vi "Main.vi"(11 "Module Admin":refnum<class "Delacor_lib_QMH_Module Admin.lvclass">) -> ()   [LabVIEW 2019, in "SME_Report.lvlib"]
doc: "This Module has below functionality.\nyou can load the csv logfile you created in the last\nstep and make the following calculations: maximum viscosity, minimum viscosity,\naverage viscosity, standard deviation of the viscosity"
uses:
  SME_Report.lvlib
  <vilib>/Delacor/Delacor QMH/Libraries/Module Admin_class/Delacor_lib_QMH_Module Admin.lvclass
  Module Data--cluster.ctl
  <vilib>/Delacor/Delacor QMH/Libraries/Message Queue_class/Delacor_lib_QMH_Message Queue.lvclass/Delacor_lib_QMH_Message Queue.ctl
  Stop Argument--cluster.ctl
  <vilib>/Delacor/Delacor QMH/Libraries/Module Admin_class/Delacor_lib_QMH_Module Admin.lvclass/Delacor_lib_QMH_Module Admin.ctl
  <vilib>/Delacor/Delacor QMH/Libraries/Message Queue_class/Delacor_lib_QMH_Enqueue Message (Single).vi
  <vilib>/Delacor/Delacor QMH/Libraries/Module Admin_class/Delacor_lib_QMH_Get External Launch.vi
  <vilib>/Delacor/Delacor QMH/Libraries/Message Queue_class/Delacor_lib_QMH_Message Queue.lvclass
panel:
  in  "Close":bool
  out "Calculation":T1 {"SD" format="%.3f"; "AVG" format="%.3f"; "Min" format="%.3f"; "Max" format="%.3f"}
  in  "Calc":bool
  in  "Path":path caption="File Path"
  out "error out":errorcluster
  out "Status":string
  in  "Simulate MHL Error":bool
  in  "Simulate EHL Error":bool
  # "Data Analysis"
  # "Other processes communicate with this Module via its Public API (wrappers for its Request Events).\n\nThis Module communicates with other processes via its Broadcast Events.\nAny process that wants to receive these messages can register for this module's Broadcast events."
  # "This template is for the DQMH framework. See the block diagram for more information on how to use this template."
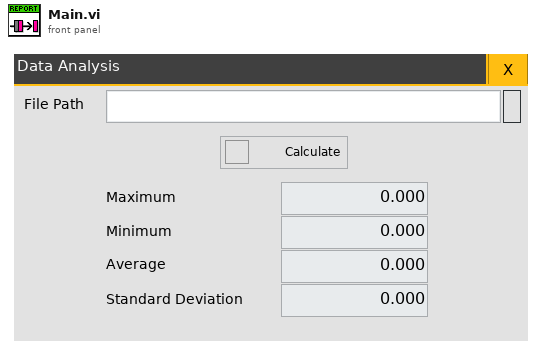
[diagram p1: front panel]
types:
  T1 = cluster{"Max":dbl, "Min":dbl, "AVG":dbl, "SD":dbl}
  T2 = typedef "SME_Report.lvlib/Request Events--cluster.ctl" = cluster{"Stop Module":refnum<user-event>, "Show Panel":refnum<user-event>, "Hide Panel":refnum<user-event>, "Get Module Execution Status":refnum<user-event>, "Show Diagram":refnum<user-event>}
  T3 = typedef "SME_Report.lvlib/Module Data--cluster.ctl" = cluster{"Status":string}
  T4 = enum32{"invalid lock state", "Not Locked", "Locked (No Password)", "Password-protected"}
  T5 = typedef "SME_Report.lvlib/Stop Argument--cluster.ctl" = cluster{"Origin":string, "Exit via Stop Module Req?":bool, "Wait for Module to stop?":bool}
  T6 = enum32{"Invalid", "Standard", "Closed", "Hidden", "Minimized", "Maximized"}
  T7 = cluster{"[0]":dbl, "[1]":dbl, "[2]":dbl, "[3]":dbl}
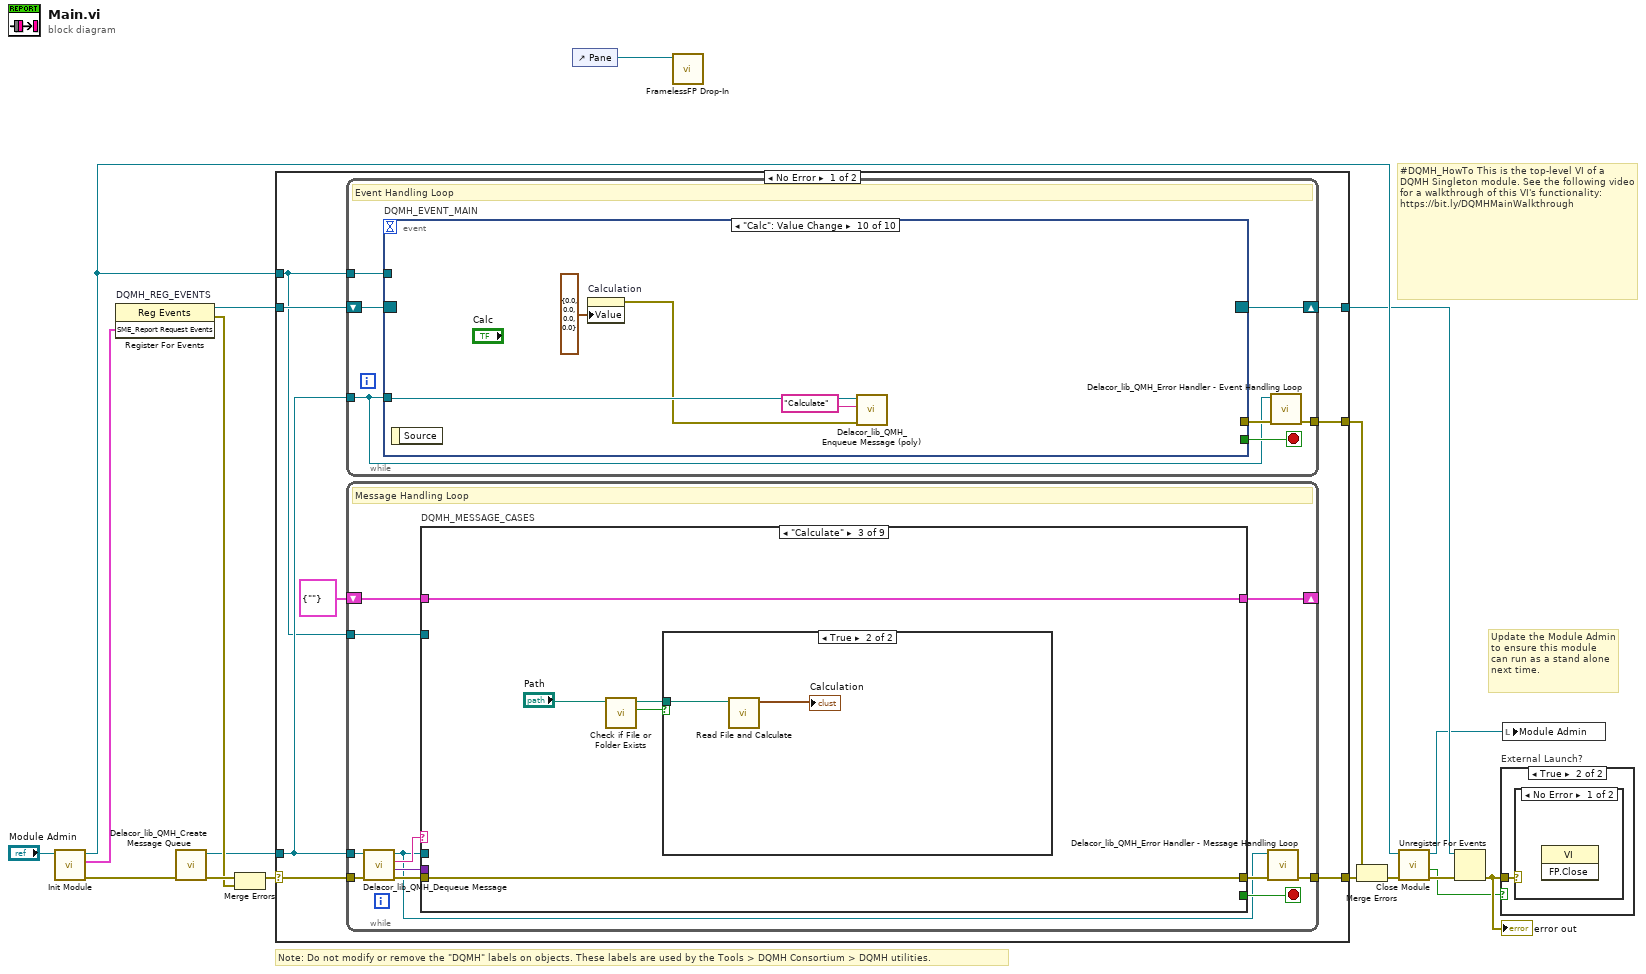
[diagram p0: block diagram]
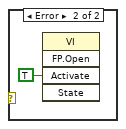
[diagram p3: hidden frame]
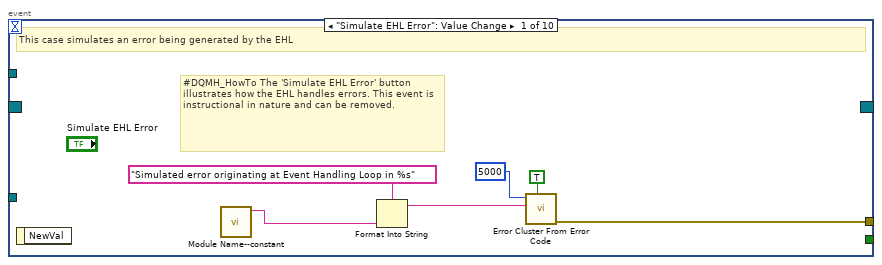
[diagram p4: hidden frame]
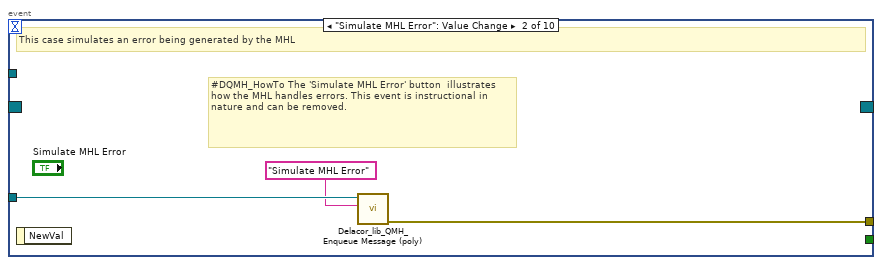
[diagram p5: hidden frame]
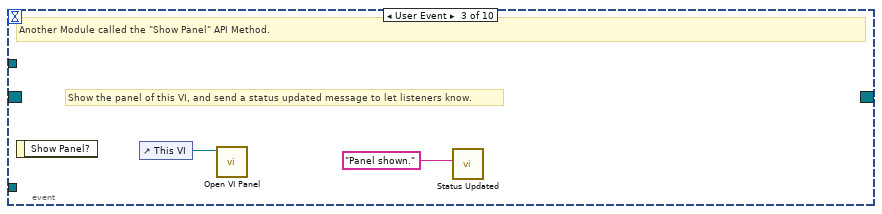
[diagram p6: hidden frame]
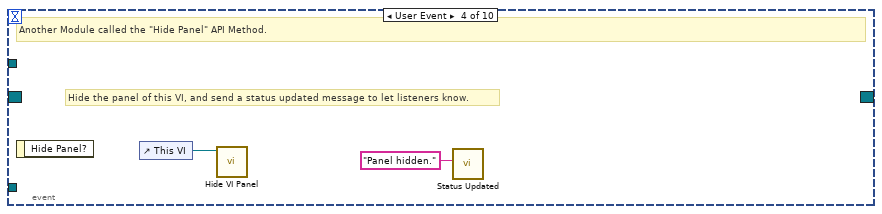
[diagram p7: hidden frame]
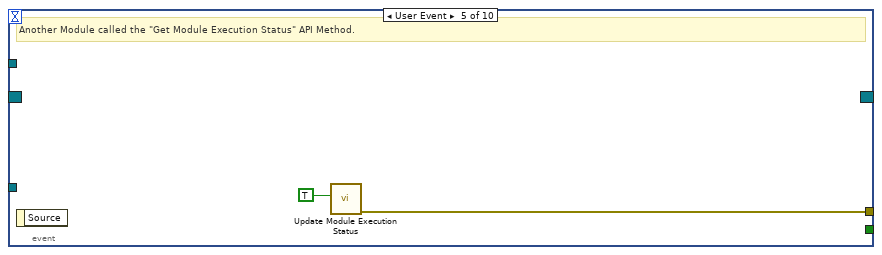
[diagram p8: hidden frame]
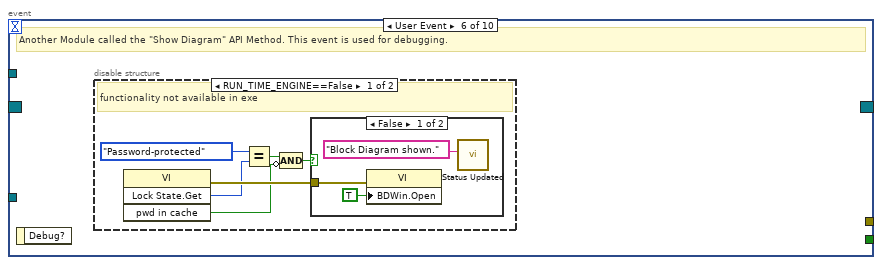
[diagram p9: hidden frame]
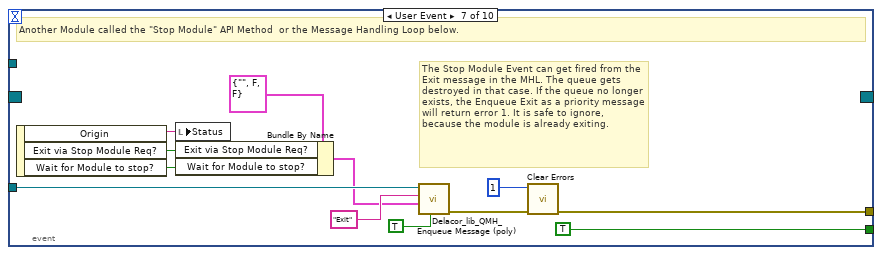
[diagram p12: hidden frame]
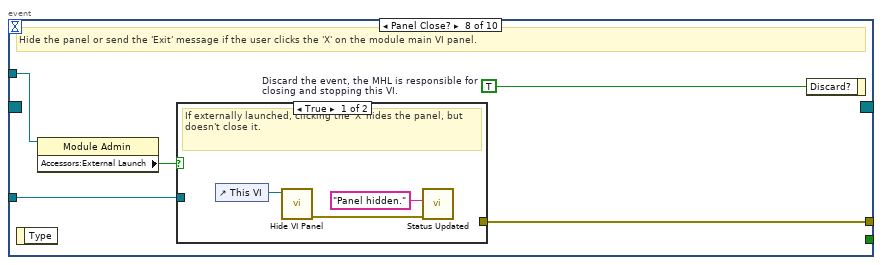
[diagram p13: hidden frame]
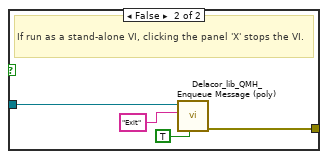
[diagram p14: hidden frame]
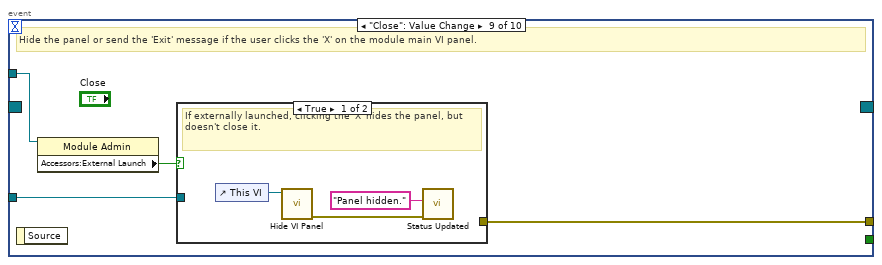
[diagram p15: hidden frame]
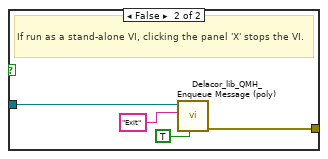
[diagram p16: hidden frame]
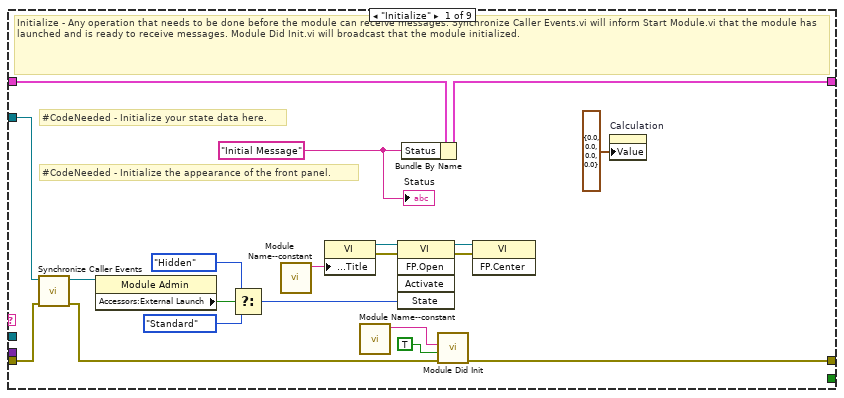
[diagram p17: hidden frame]
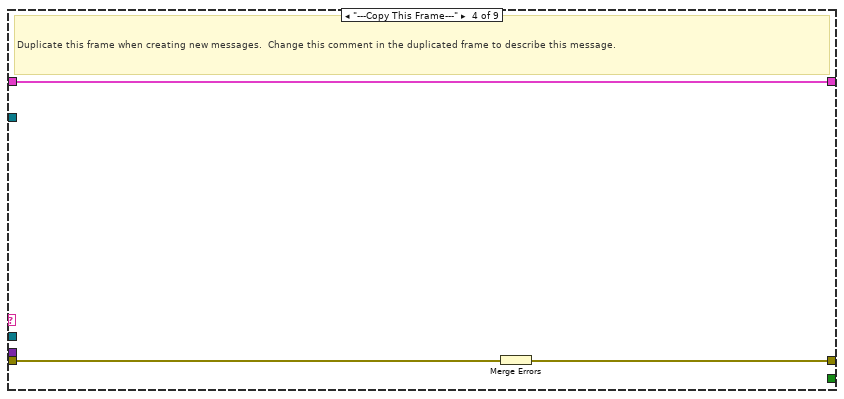
[diagram p20: hidden frame]
diagram:
  # "#DQMH_HowTo This is the top-level VI of a DQMH Singleton module. See the following video for a walkthrough of this VI's functionality: https://bit.ly/DQMHMainWalkthrough"
  # "Note: Do not modify or remove the \"DQMH\" labels on objects. These labels are used by the Tools > DQMH Consortium > DQMH utilities."
  # "Update the Module Admin to ensure this module can run as a stand alone next time."
  n1 = call "Init Module.vi"("Singleton Module Admin in"="Module Admin") -> ("error out"=w17:errorcluster, "SME_Report Request Events"=w6:T2, "Singleton Module Admin out"=w9:refnum<class "Delacor_lib_QMH_Module Admin.lvclass">)  [unwired: 8 in]
  n2 = register-events "DQMH_REG_EVENTS"(w6) -> (reference out=w7:refnum<event-registration>, error out=w10:errorcluster)  [unwired: 2 in]
  n3 = call <vilib>:"Delacor_lib_QMH_Create Message Queue.vi"("error in"=w17) -> ("error out"=w12:errorcluster, "Message Queue"=w5:refnum<class "Delacor_lib_QMH_Message Queue.lvclass">)  [unwired: 9 in]
  n4 = Merge Errors(w12, w10) -> (w11:errorcluster)
  n5 = case shown="No Error" w11 {
    selector: w11 -> [w24 w201]
    tunnel: [w26 w200] -> w18
    tunnel: [w23 w199] -> w8
    tunnel: w7 -> [w21 w199]
    tunnel: w5 -> [w20 w194]
    tunnel: [w25 _] -> w15
    tunnel: w9 -> [w19 w195]
    frame No Error {
      n6 = while {
        tunnel: w20 -> [w27]
        shift-right: [w30] -> w23
        shift-left: w21 -> [w31]
        tunnel: [w32] -> w25
        tunnel: w19 -> [w28]
        stop <- w29 stop-if-true
        # "Event Handling Loop"
        n7 = event "DQMH_EVENT_MAIN" shown="[9] \"Calc\": Value Change" {
          selector: w31 -> [_ _ _ _ _ _ _ _ _ _]
          dyn-events: [_ _ _ _ _ _ _ _ _ _] -> w30
          timeout: _ -> [_ _ _ _ _ _ _ _ _ _]
          tunnel: [_ _ _ _ _ _ TRUE ("Discard?") _ _ _] -> w29
          tunnel: w27 -> [_ w41 _ _ _ _ w65 w72 w84 w95]
          tunnel: [w39 w42 _ _ w48 _ w68 w74 w85 _] -> w33
          tunnel: w28 -> [_ _ _ _ _ _ _ w71 w83 _]
          event "Simulate EHL Error": Value Change {
            # "#DQMH_HowTo The 'Simulate EHL Error' button  illustrates how the EHL handles errors. This event is instructional in nature and can be removed."
            # "This case simulates an error being generated by the EHL"
            n8 = event-data() -> ()  [unwired: 1 in, 1 out]
            n9 = call "Module Name--constant.vi"() -> ("Module Name"=w36:string)  [unwired: 11 in]
            n10 = Format Into String(format string="Simulated error originating at Event Handling Loop in %s", w36) -> (resulting string=w37:string)  [unwired: 2 in, 1 out]
            n11 = call <vilib>:"Error Cluster From Error Code.vi"("show call chain? (False)"=TRUE, "error message (\"\")"=w37, "error code (0)"=5000) -> ("error out"=w39:errorcluster)  [unwired: 6 in]
          }
          event "Simulate MHL Error": Value Change {
            # "#DQMH_HowTo The 'Simulate MHL Error' button  illustrates how the MHL handles errors. This event is instructional in nature and can be removed."
            # "This case simulates an error being generated by the MHL"
            n12 = event-data() -> ()  [unwired: 1 in, 1 out]
            n13 = call-poly <vilib>:"Delacor_lib_QMH_Enqueue Message (poly).vi"("Message"="Simulate MHL Error", "Message Queue in"=w41) -> ("error out"=w42:errorcluster)  [unwired: 8 in, 1 out]
          }
          event User Event {
            # "Show the panel of this VI, and send a status updated message to let listeners know."
            # "Another Module called the \"Show Panel\" API Method."
            n14 = event-data() -> ()  [unwired: 1 in, 1 out]
            n15 = control-ref of="This VI"() -> (w44:refnum<vi>)
            n16 = call "Open VI Panel.vi"("VI"=w44) -> ()  [unwired: 10 in, 1 out]
            n17 = call "Status Updated.vi"("Status"="Panel shown." ("format string")) -> ()  [unwired: 10 in, 1 out]
          }
          event User Event {
            # "Hide the panel of this VI, and send a status updated message to let listeners know."
            # "Another Module called the \"Hide Panel\" API Method."
            n18 = event-data() -> ()  [unwired: 1 in, 1 out]
            n19 = control-ref of="This VI"() -> (w46:refnum<vi>)
            n20 = call "Hide VI Panel.vi"("VI"=w46) -> ()  [unwired: 10 in, 1 out]
            n21 = call "Status Updated.vi"("Status"="Panel hidden." ("format string")) -> ()  [unwired: 10 in, 1 out]
          }
          event User Event {
            # "Another Module called the \"Get Module Execution Status\" API Method."
            n22 = event-data() -> ()  [unwired: 1 in, 1 out]
            n23 = call "Update Module Execution Status.vi"("Running?"=TRUE) -> ("error out"=w48:errorcluster)  [unwired: 10 in]
          }
          event User Event {
            # "Another Module called the \"Show Diagram\" API Method. This event is used for debugging."
            n24 = event-data() -> ()  [unwired: 1 in, 1 out]
            n25 = disable-structure shown="RUN_TIME_ENGINE==False" {
              frame condition #0 (active) {
                # "functionality not available in exe"
                n26 = invoke on="Invoke Node" class="VI" method="Lock State.Get"() -> (error out=w54:errorcluster, "Get Lock State"=w53:T4, "pwd in cache"=w50:bool)  [unwired: 4 in, 1 out]
                n27 = Equal?(x=T4."Password-protected", y=w53) -> (x = y?=w51:bool)
                n28 = Compound Arithmetic op=AND(w51, invert w50) -> (w49:bool)
                n29 = case shown="False" w49 {
                  tunnel: w54 -> [w57 _]
                  frame False {
                    n30 = property on="Property Node" class="VI"(error in=w57, "BDWin.Open"=TRUE ("Block Diagram Window:Open")) -> ()  [unwired: 1 in, 2 out]
                    n31 = call "Status Updated.vi"("Status"="Block Diagram shown." ("format string")) -> ()  [unwired: 10 in, 1 out]
                  }
                  frame True {
                    # "Password-protected VI, and the password is not in the cache. Do not show the diagram."
                  }
                }
              }
              frame condition #1 {
              }
            }
          }
          event User Event {
            # "The Stop Module Event can get fired from the Exit message in the MHL. The queue gets destroyed in that case. If the queue no longer exists, the Enqueue Exit as a priority message will return error 1. It is safe to ignore, because the module is already exiting."
            # "Another Module called the \"Stop Module\" API Method  or the Message Handling Loop below."
            n32 = event-data() -> ("Origin"=w64:string, "Exit via Stop Module Req?"=w60:bool, "Wait for Module to stop?"=w59:bool)  [unwired: 1 in]
            n33 = local write "Status"(w64) -> ()
            n34 = Bundle By Name(cluster=T5 {"Origin"="", "Exit via Stop Module Req?"=FALSE, "Wait for Module to stop?"=FALSE} ("Stop Argument"), "Exit via Stop Module Req?"=w60, "Wait for Module to stop?"=w59) -> (w58:T5)
            n35 = call-poly <vilib>:"Delacor_lib_QMH_Enqueue Message (poly).vi"("Priority Message? (F)"=TRUE, "Message Data"=w58, "Message"="Exit", "Message Queue in"=w65) -> ("error out"=w69:errorcluster)  [unwired: 6 in, 1 out]
            n36 = call <vilib>:"Clear Errors.vi"("error in (no error)"=w69, "specific error code to clear (0: all)"=1) -> ("error out"=w68:errorcluster)  [unwired: 4 in, 1 out]
          }
          event Panel Close? {
            w73 = TRUE  # Discard the event, the MHL is responsible for closing and stopping this VI.
            # "Hide the panel or send the 'Exit' message if the user clicks the 'X' on the module main VI panel."
            n37 = event-data() -> ()  [unwired: 1 in, 1 out]
            n38 = property on="Property Node" class="Module Admin"(reference=w71) -> ("Accessors:External Launch"=w70:bool)  [unwired: 1 in, 2 out]
            n39 = case shown="True" w70 {
              tunnel: w72 -> [_ w80]
              tunnel: [_ w81] -> w74
              frame True {
                # "If externally launched, clicking the 'X' hides the panel, but doesn't close it."
                n40 = control-ref of="This VI"() -> (w77:refnum<vi>)
                n41 = call "Hide VI Panel.vi"("VI"=w77) -> ("error out"=w75:errorcluster)  [unwired: 10 in]
                n42 = call "Status Updated.vi"("error in"=w75, "Status"="Panel hidden." ("format string")) -> ()  [unwired: 9 in, 1 out]
              }
              frame False {
                # "If run as a stand-alone VI, clicking the panel 'X' stops the VI."
                n43 = call-poly <vilib>:"Delacor_lib_QMH_Enqueue Message (poly).vi"("Priority Message? (F)"=TRUE, "Message"="Exit", "Message Queue in"=w80) -> ("error out"=w81:errorcluster)  [unwired: 7 in, 1 out]
              }
            }
            n44 = event-data ("Event Filter Node")("Discard?"=w73) -> ()  [unwired: 1 in, 1 out]
          }
          event "Close": Value Change {
            # "Hide the panel or send the 'Exit' message if the user clicks the 'X' on the module main VI panel."
            n45 = event-data() -> ()  [unwired: 1 in, 1 out]
            n46 = property on="Property Node" class="Module Admin"(reference=w83) -> ("Accessors:External Launch"=w82:bool)  [unwired: 1 in, 2 out]
            n47 = case shown="True" w82 {
              tunnel: w84 -> [_ w91]
              tunnel: [_ w92] -> w85
              frame True {
                # "If externally launched, clicking the 'X' hides the panel, but doesn't close it."
                n48 = control-ref of="This VI"() -> (w88:refnum<vi>)
                n49 = call "Hide VI Panel.vi"("VI"=w88) -> ("error out"=w86:errorcluster)  [unwired: 10 in]
                n50 = call "Status Updated.vi"("error in"=w86, "Status"="Panel hidden." ("format string")) -> ()  [unwired: 9 in, 1 out]
              }
              frame False {
                # "If run as a stand-alone VI, clicking the panel 'X' stops the VI."
                n51 = call-poly <vilib>:"Delacor_lib_QMH_Enqueue Message (poly).vi"("Priority Message? (F)"=TRUE, "Message"="Exit", "Message Queue in"=w91) -> ("error out"=w92:errorcluster)  [unwired: 7 in, 1 out]
              }
            }
          }
          event "Calc": Value Change {
            n52 = event-data() -> ()  [unwired: 1 in, 1 out]
            n53 = property on="Calculation" class="Clust (strict)"("Value"=T1 {"Max"=0.0, "Min"=0.0, "AVG"=0.0, "SD"=0.0} ("Calculation")) -> (error out=w93:errorcluster)  [unwired: 2 in, 1 out]
            n54 = call-poly <vilib>:"Delacor_lib_QMH_Enqueue Message (poly).vi"("error in"=w93, "Message"="Calculate", "Message Queue in"=w95) -> ()  [unwired: 7 in, 2 out]
          }
        }
        n55 = call-dynamic "Delacor_lib_QMH_Error Handler - Event Handling Loop.vi"("error in"=w33, "Message Queue in"=w27) -> ("dup error in"=w32:errorcluster)  [unwired: 8 in, 1 out]
      }
      n56 = while {
        tunnel: w20 -> [w97]
        shift-right: [w105] -> _
        shift-left: T3 {"Status"=""} ("Data Cluster") -> [w106]
        tunnel: w24 -> [w108]
        tunnel: [w100] -> w26
        tunnel: w19 -> [w101]
        stop <- w104 stop-if-true
        # "Message Handling Loop"
        n57 = call-dynamic "Delacor_lib_QMH_Dequeue Message.vi"("error in"=w108, "Message Queue in"=w97) -> ("error out"=w107:errorcluster, "Message Data"=w102:variant, "Message"=w103:string, "Message Queue out"=w98:refnum<class "Delacor_lib_QMH_Message Queue.lvclass">)  [unwired: 6 in]
        n58 = case "DQMH_MESSAGE_CASES" shown="\"Calculate\"" w103 {
          selector: w103 -> [_ _ _ _ _ _ _ _ w189]
          tunnel: w98 -> [_ _ _ _ _ _ w155 w177 _]
          tunnel: w107 -> [w126 w130 w135 w140 w142 w151 w162 w183 w192]
          tunnel: [w124 w130 w135 w139 w142 w150 w158 w178 w193] -> w99
          tunnel: w106 -> [w115 w129 w134 w138 w141 w148 w157 w176 w190]
          tunnel: [w114 w129 w134 w138 w141 w148 w157 w176 w190] -> w105
          tunnel: [_ _ _ _ _ _ _ w175 _] -> w104
          tunnel: w102 -> [_ _ _ _ _ _ w156 w174 _]
          tunnel: w101 -> [w116 _ _ _ _ _ w154 w169 _]
          frame "Initialize" {
            w110 = "Initial Message" ("Initial Message")
            # "#CodeNeeded - Initialize the appearance of the front panel."
            # "#CodeNeeded - Initialize your state data here."
            # "Initialize - Any operation that needs to be done before the module can receive messages. Synchronize Caller Events.vi will inform Start Module.vi that the module has launched and is ready to receive messages. Module Did Init.vi will broadcast that the module initialized."
            n59 = call "Synchronize Caller Events.vi"("error in"=w126, "Singleton Module Admin in"=w116) -> ("error out"=w125:errorcluster, "Singleton Module Admin out"=w111:refnum<class "Delacor_lib_QMH_Module Admin.lvclass">)  [unwired: 8 in]
            n60 = property on="Property Node" class="Module Admin"(reference=w111) -> ("Accessors:External Launch"=w120:bool)  [unwired: 1 in, 2 out]
            n61 = Select(t=T6."Hidden" ("State"), s=w120, f=T6."Standard" ("State")) -> (s? t:f=w117:T6)
            n62 = call "Module Name--constant.vi"() -> ("Module Name"=w123:string)  [unwired: 11 in]
            n63 = property on="Property Node" class="VI"("Front Panel.Title"=w123) -> (reference out=w122:refnum<vi>, error out=w128:errorcluster)  [unwired: 2 in]
            n64 = call "Module Name--constant.vi"() -> ("Module Name"=w112:string)  [unwired: 11 in]
            n65 = invoke on="Invoke Node" class="VI" method="FP.Open"(reference=w122, error in=w128, "State"=w117) -> (reference out=w121:refnum<vi>, error out=w127:errorcluster)  [unwired: 2 in, 3 out]
            n66 = Bundle By Name(cluster=w115, "Status"=w110) -> (w114:T3)
            n67 = call "Module Did Init.vi"("error in"=w125, "Initialized?"=TRUE, "Origin"=w112) -> ("error out"=w124:errorcluster)  [unwired: 8 in]
            n68 = invoke on="Invoke Node" class="VI" method="FP.Center"(reference=w121, error in=w127) -> ()  [unwired: 1 in, 3 out]
            n69 = property on="Calculation" class="Clust (strict)"("Value"=T1 {"Max"=0.0, "Min"=0.0, "AVG"=0.0, "SD"=0.0} ("Calculation")) -> ()  [unwired: 2 in, 2 out]
            "Status" <- w110
          }
          frame "---Module Specific---" {
            # "Separator -- The following cases handle messages specific to this Module."
          }
          frame "Calculate" {
            n70 = call <vilib>:"Check if File or Folder Exists.vi"("path"="Path") -> ("file or folder exists?"=w132:bool, "dup path"=w131:path)  [unwired: 8 in, 1 out]
            n71 = case shown="True" w132 {
              tunnel: w131 -> [_ w137]
              frame False {
              }
              frame True {
                n72 = call "Read File and Calculate.vi"("file path (dialog if empty)"=w137) -> ("Cluster"=→"Calculation":T7)  [unwired: 10 in]
              }
            }
          }
          frame "---Copy This Frame---" {
            # "Duplicate this frame when creating new messages.  Change this comment in the duplicated frame to describe this message."
            n73 = Merge Errors(w140) -> (w139:errorcluster)
          }
          frame "---Exit and Error Handling---" {
            # "Separator - The following cases handle errors and exit messages."
          }
          frame "Simulate MHL Error" {
            # "#DQMH_HowTo The 'Simulate MHL Error' button  illustrates how the MHL handles errors. This event is instructional in nature and can be removed."
            # "Simulate an error occurring at the MHL"
            n74 = call "Module Name--constant.vi"() -> ("Module Name"=w144:string)  [unwired: 11 in]
            n75 = Format Into String(format string="Simulated error originating at Message Handling Loop in %s", w144) -> (resulting string=w145:string)  [unwired: 2 in, 1 out]
            n76 = call <vilib>:"Error Cluster From Error Code.vi"("show call chain? (False)"=TRUE, "error message (\"\")"=w145, "error code (0)"=5001) -> ("error out"=w149:errorcluster)  [unwired: 6 in]
            n77 = Merge Errors(w151, w149) -> (w150:errorcluster)
          }
          frame "Error" {
            # "#CodeRecommended - If the module is running in standalone mode (External Launch = FALSE), this code will pop up an error dialog and call the 'Exit' message if an error occurs. Add more fine-grained error management here."
            # "Error - Check the error message data and respond accordingly. This message is sent by the \"Error Handler\" VIs at the end of each loop in this application."
            n78 = property on="Property Node" class="Module Admin"(reference=w154) -> ("Accessors:External Launch"=w153:bool)  [unwired: 1 in, 2 out]
            n79 = Variant To Data(error in=w162, type=errorcluster {"status"=FALSE, "code"=0, "source"=""} ("error constant"), Variant=w156) -> (data=w152:errorcluster, error out=w160:errorcluster)
            n80 = local write "error out"(w152) -> ()
            n81 = call "Error Reported.vi"("Error"=w152) -> ()  [unwired: 10 in, 1 out]
            n82 = case shown="False" w153 {
              tunnel: [w167 _] -> w159
              tunnel: w155 -> [w165 _]
              tunnel: w152 -> [w166 _]
              frame False {
                n83 = disable-structure shown="Default" {
                  disable-tunnel: w166 -> [w168 _]
                  frame condition #0 (active) {
                    # "If the module is running standalone, then pop up an error dialog and call the \"Exit\" message."
                    n84 = call <vilib>:"Simple Error Handler.vi"("error in (no error)"=w168) -> ()  [unwired: 4 in, 5 out]
                  }
                  frame condition #1 {
                    # "To prevent the Simple Error Handler VI from being loaded (e.g. when deploying to a Real-Time target), add the Conditional Disable Symbol \"DQMH_Disable_SEH\" to your project and set it to TRUE."
                  }
                }
                n85 = call-poly <vilib>:"Delacor_lib_QMH_Enqueue Message (poly).vi"("Priority Message? (F)"=TRUE, "Message"="Exit", "Message Queue in"=w165) -> ("error out"=w167:errorcluster)  [unwired: 7 in, 1 out]
              }
              frame True {
                # "If the module was launched externally, calling the Error Reported broadcast VI is the only action performed by the \"Error\" message. The module's caller can then process the error appropriately."
              }
            }
            n86 = Merge Errors(w160, w159) -> (w158:errorcluster)
          }
          frame "Exit" {
            w173 = 91  # 91: not all Exit messages will have an argument
            w175 = TRUE  # Stop the VI
            # "Release the message queue reference"
            # "#CodeNeeded - Add any required cleanup code here."
            # "Exit - Exit the application."
            n87 = Variant To Data(error in=w183, type=T5 {"Origin"="", "Exit via Stop Module Req?"=FALSE, "Wait for Module to stop?"=FALSE} ("Stop Argument"), Variant=w174) -> (data=w171:T5, error out=w180:errorcluster)
            n88 = call <vilib>:"Clear Errors.vi"("error in (no error)"=w180, "specific error code to clear (0: all)"=w173) -> ("error out"=w182:errorcluster)  [unwired: 4 in, 1 out]
            n89 = control-ref of="This VI"() -> (w170:refnum<vi>)
            n90 = call-dynamic "Delacor_lib_QMH_Release Message Queue.vi"("error in"=w182, "Message Queue"=w177) -> ("error out"=w181:errorcluster)  [unwired: 9 in]
            n91 = call "Handle Exit.vi"("Stop Argument"=w171, "Admin in"=w169, "VI reference"=w170) -> ("error out"=w179:errorcluster)  [unwired: 7 in, 1 out]
            n92 = Merge Errors(w181, w179) -> (w178:errorcluster)
            n93 = call "Error Reported.vi"("Error"=w178) -> ()  [unwired: 10 in, 1 out]
          }
          frame Default {
            # "'Default' case only runs if there is a message that isn't defined in any of the other cases.  Output a programming error."
            n94 = call "Module Name--constant.vi"() -> ("Module Name"=w188:string)  [unwired: 11 in]
            n95 = Format Into String(format string="The invalid message string \"%s\" was received in the Message Handling Loop for module \"%s\".", w189, w188) -> (resulting string=w184:string)  [unwired: 2 in, 1 out]
            n96 = call <vilib>:"Error Cluster From Error Code.vi"("show call chain? (False)"=TRUE, "error message (\"\")"=w184, "error code (0)"=1) -> ("error out"=w191:errorcluster)  [unwired: 6 in]
            n97 = Merge Errors(w192, w191) -> (w193:errorcluster)
          }
        }
        n98 = call-dynamic "Delacor_lib_QMH_Error Handler - Message Handling Loop.vi"("error in"=w99, "Message Queue in"=w98) -> ("dup error in"=w100:errorcluster)  [unwired: 8 in, 1 out]
      }
    }
    frame Error {
      # "Synchronize Caller Events.vi will inform Start Module.vi that the module has launched and will let the code calling Start Module.vi register for broadcasts and would permit the caller receive the broadcast that an error occurred at launch time."
      n99 = call-dynamic "Delacor_lib_QMH_Release Message Queue.vi"("error in"=w201, "Message Queue"=w194) -> ("error out"=w200:errorcluster)  [unwired: 9 in]
      n100 = call "Synchronize Caller Events.vi"("Singleton Module Admin in"=w195) -> ("error out"=w202:errorcluster)  [unwired: 9 in, 1 out]
      n101 = call "Module Name--constant.vi"() -> ("Module Name"=w198:string)  [unwired: 11 in]
      n102 = Format Into String(format string="An error occurred during initialization. %s is no longer running.", w198) -> (resulting string=w196:string)  [unwired: 2 in, 1 out]
      n103 = Merge Errors(w200, w202) -> (w203:errorcluster)
      n104 = call "Error Reported.vi"("Additional Information"=w196, "Error"=w203) -> ()  [unwired: 9 in, 1 out]
    }
  }
  n105 = control-ref of="Pane"() -> (w1:refnum<vi>)
  n106 = call "FramelessFP Drop-In.vi"("Pane in"=w1) -> ()  [unwired: 10 in, 1 out]
  n107 = Merge Errors(w15, w18) -> (w14:errorcluster)
  n108 = call "Close Module.vi"("error in"=w14, "Module Admin in"=w9) -> ("error out"=w16:errorcluster, "External Launch"=w2:bool, "Module Admin out"=w3:refnum<class "Delacor_lib_QMH_Module Admin.lvclass">)  [unwired: 7 in]
  n109 = Unregister For Events(event registration refnum=w8, error in=w16) -> (error out=w13:errorcluster)
  "error out" <- w13
  n110 = case "External Launch?" shown="True" w2 {
    tunnel: w13 -> [_ w204]
    frame False {
    }
    frame True {
      n111 = case shown="No Error" w204 {
        frame No Error {
          n112 = invoke on="Invoke Node" class="VI" method="FP.Close"() -> ()  [unwired: 3 in, 3 out]
        }
        frame Error {
          n113 = invoke on="Invoke Node" class="VI" method="FP.Open"("Activate"=TRUE ("Activate?")) -> ()  [unwired: 4 in, 5 out]
        }
      }
    }
  }
  n114 = local write "Module Admin"(w3) -> ()
